vi "Periodic Tasks.vi"(8 "error in":errorcluster) -> ()   [LabVIEW 2018]
doc: "This VI runs in parallel to other robot code. It can contain as many user-defined periodic loops as you need. These can carry out PID or other sorts of timed response."
uses:
  <vilib>/Rock Robotics/WPI/Utilities/WPI_GetSetVariantRefNum.vi
  Robot Global Data.vi
  <vilib>/Rock Robotics/Network Tables/NT Read Number.vi
  <vilib>/Rock Robotics/Network Tables/NT Read String.vi
panel:
  out "Y Position":dbl min=-1.0 max=1.0 step=0.1 format="%#_2f"
  out "X Position":dbl min=-1.0 max=1.0 step=0.1 format="%#_2f"
  out "Intake Speed":dbl min=-1.0 max=1.0 step=0.1 format="%#_2f"
  out "Shooter Speed":dbl min=-1.0 max=1.0 step=0.1 format="%#_2f"
  out "Autonomous Sequence":string
  out "Drive type":i8
  out "Drive Number":i8
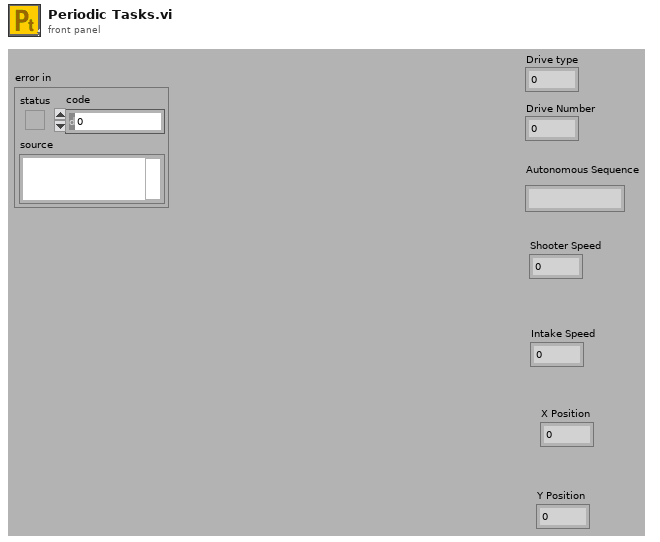
[diagram p1: front panel]
types:
  T1 = typedef "WPI_MotorControlDeviceRef.ctl" = cluster{"DeviceStatus":errorcluster, "Type":T2, "PWM":cluster{"PWM Channel":T3, "DeadBand":T4}, "CAN":cluster{"Device Number":u8, "SetOutput VI Ref":variant, "GetOutput VI Ref":variant, "Enable VI Ref":variant, "Disable VI Ref":variant, "Data":variant}, "Invert":bool, "DIO PWM":cluster{"PWM \"Enable\" Channel":T3, "DIOChannel":T5, "PWM Rate":dbl}}
  T2 = typedef "WPI_MotorControlType.ctl" = enum16{"PWM", "CAN", "DIO PWM"}
  T3 = typedef "FPGA_DIOPWMChannel.ctl" = enum8{"PWM 0", "PWM 1", "PWM 2", "PWM 3", "PWM 4", "PWM 5", "PWM 6", "PWM 7", "PWM 8", "PWM 9", "PWM MXP 0", "PWM MXP 1", "PWM MXP 2", "PWM MXP 3", "PWM MXP 4", "PWM MXP 5", "PWM MXP 6", "PWM MXP 7", "PWM MXP 8", "PWM MXP 9", "Invalid"}
  T4 = typedef "WPI_PWMDeadband.ctl" = cluster{"Name":string, "maxPositivePwm":i32, "minPositivePwm":i32, "centerPwm":i32, "maxNegativePwm":i32, "minNegativePwm":i32, "angularRange":u16}
  T5 = typedef "FPGA_DIOChannel.ctl" = enum8{"DIO 0", "DIO 1", "DIO 2", "DIO 3", "DIO 4", "DIO 5", "DIO 6", "DIO 7", "DIO 8", "DIO 9", "DIO MXP 0", "DIO MXP 1", "DIO MXP 2", "DIO MXP 3", "DIO MXP 4", "DIO MXP 5", "DIO MXP 6", "DIO MXP 7", "DIO MXP 8", "DIO MXP 9", "DIO MXP 10", "DIO MXP 11", "DIO MXP 12", "DIO MXP 13", "DIO MXP 14", "DIO MXP 15", "SPI Port CS1", "SPI Port CS2", "SPI Port CS3", "SPI Port MISO", "SPI Port MOSI", "Invalid"}
  T6 = typedef "WPI_JoystickDevRef.ctl" = cluster{"Device":T7}
  T7 = typedef "WPI_JoystickDeviceEnum.ctl" = enum16{"USB 0", "USB 1", "USB 2", "USB 3", "USB 4", "USB 5"}
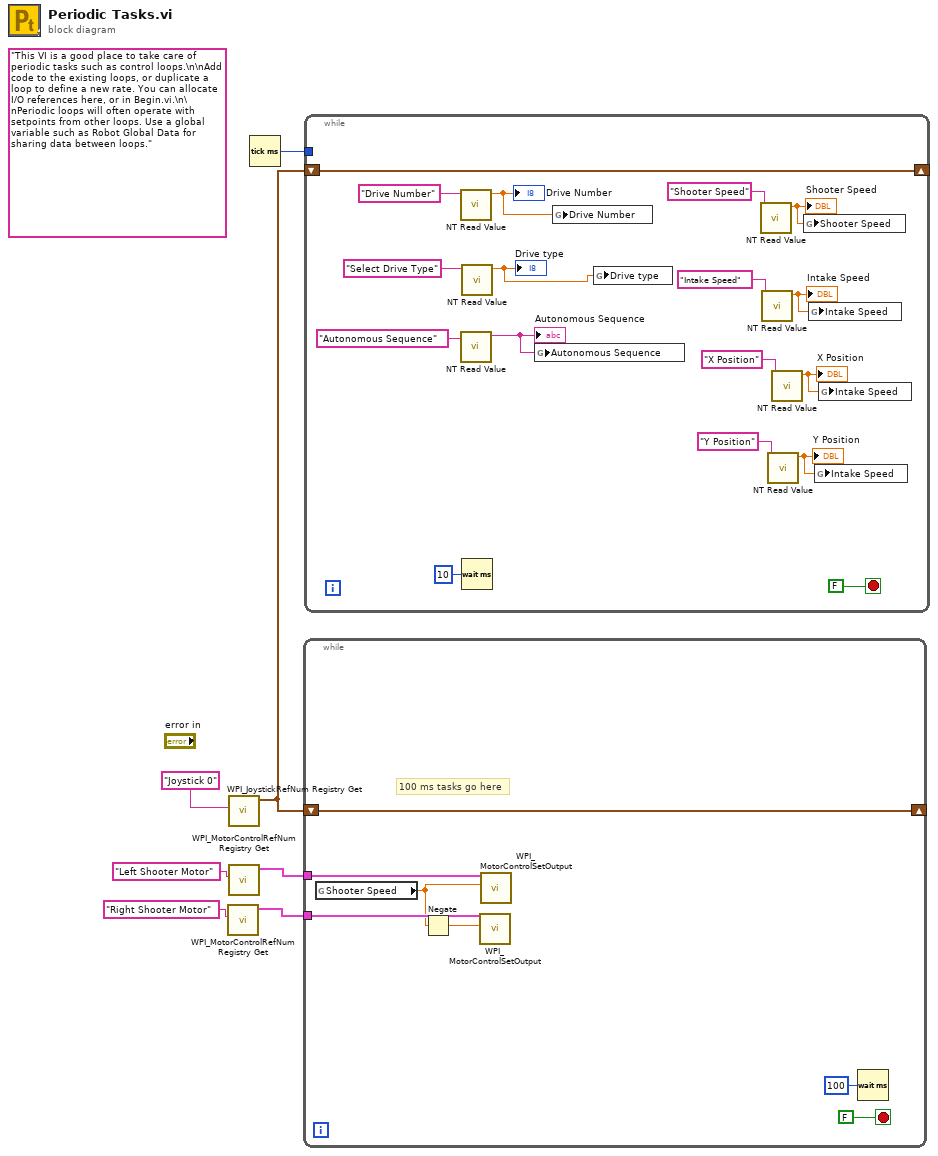
[diagram p0: block diagram]
diagram:
  (unwired) "This VI is a good place to take care of periodic tasks such as control loops.\n\nAdd code to the existing loops, or duplicate a loop to define a new rate. You can allocate I/O references here, or in Begin.vi.\n\nPeriodic loops will often operate with setpoints from other loops. Use a global variable such as Robot Global Data for sharing data between loops."
  n1 = call <vilib>:"WPI_MotorControlRefNum Registry Get.vi"("refnum name"="Right Shooter Motor") -> ("MotorControlDevRef"=w1:T1)  [unwired: 9 in, 1 out]
  n2 = call <vilib>:"WPI_JoystickRefNum Registry Get.vi"("refnum name"="Joystick 0") -> ("JoystickDevRef"=w6:T6)  [unwired: 1 in, 9 out]
  n3 = call <vilib>:"WPI_MotorControlRefNum Registry Get.vi"("refnum name"="Left Shooter Motor") -> ("MotorControlDevRef"=w2:T1)  [unwired: 9 in, 1 out]
  n4 = Tick Count (ms)() -> (millisecond timer value=w5:u32)
  n5 = while {
    shift-right: [w12] -> _
    shift-left: w6 -> [w12]
    tunnel: w2 -> [w11]
    tunnel: w1 -> [w10]
    stop <- FALSE stop-if-true
    # "100 ms tasks go here"
    n6 = global read "Robot Global Data.vi" "Shooter Speed"() -> (w9:dbl)
    n7 = Negate(x=w9) -> (-x=w8:dbl)
    n8 = call <vilib>:"WPI_MotorControlSetOutput.vi"("Output"=w8, "MotorControlDevRef"=w10) -> ()  [unwired: 7 in, 3 out]
    n9 = call <vilib>:"WPI_MotorControlSetOutput.vi"("Output"=w9, "MotorControlDevRef"=w11) -> ()  [unwired: 7 in, 3 out]
    n10 = Wait (ms)(milliseconds to wait=u32 100) -> ()  [unwired: 1 out]
  }
  n11 = while {
    shift-right: [w30] -> _
    shift-left: w6 -> [w30]
    tunnel: w5 -> [_]
    stop <- FALSE stop-if-true
    n12 = call-poly <vilib>:"NT Read Value.vi"("Name"="Drive Number") -> ("Numeric"=w24:dbl)  [unwired: 9 in, 1 out]
    "Drive Number" <- w24
    n13 = call-poly <vilib>:"NT Read Value.vi"("Name"="Autonomous Sequence") -> ("String"=w22:string)  [unwired: 9 in, 1 out]
    "Autonomous Sequence" <- w22
    n14 = call-poly <vilib>:"NT Read Value.vi"("Name"="Select Drive Type") -> ("Numeric"=w23:dbl)  [unwired: 9 in, 1 out]
    "Drive type" <- w23
    n15 = Wait (ms)(milliseconds to wait=u32 10) -> ()  [unwired: 1 out]
    n16 = global write "Robot Global Data.vi" "Autonomous Sequence"(w22) -> ()
    n17 = global write "Robot Global Data.vi" "Drive Number"(w24) -> ()
    n18 = global write "Robot Global Data.vi" "Drive type"(w23) -> ()
    n19 = call-poly <vilib>:"NT Read Value.vi"("Name"="Shooter Speed") -> ("Numeric"=w21:dbl)  [unwired: 9 in, 1 out]
    "Shooter Speed" <- w21
    n20 = call-poly <vilib>:"NT Read Value.vi"("Name"="Intake Speed") -> ("Numeric"=w20:dbl)  [unwired: 9 in, 1 out]
    "Intake Speed" <- w20
    n21 = call-poly <vilib>:"NT Read Value.vi"("Name"="Y Position") -> ("Numeric"=w16:dbl)  [unwired: 9 in, 1 out]
    "Y Position" <- w16
    n22 = call-poly <vilib>:"NT Read Value.vi"("Name"="X Position") -> ("Numeric"=w17:dbl)  [unwired: 9 in, 1 out]
    "X Position" <- w17
    n23 = global write "Robot Global Data.vi" "Shooter Speed"(w21) -> ()
    n24 = global write "Robot Global Data.vi" "Intake Speed"(w20) -> ()
    n25 = global write "Robot Global Data.vi" "Intake Speed"(w16) -> ()
    n26 = global write "Robot Global Data.vi" "Intake Speed"(w17) -> ()
  }
